vi "in_diff and divided diff.vi"   [LabVIEW 2020, in "NI_Gmath.lvlib"]
uses:
  <vilib>/gmath/NI_Gmath.lvlib
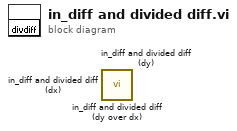
[diagram p0: block diagram]
diagram:
  n1 = call <vilib>:"in_diff and divided diff (dy over dx).vi"() -> ()  [unwired: 15 in, 1 out]
  n2 = call <vilib>:"in_diff and divided diff (dy).vi"() -> ()  [unwired: 15 in, 1 out]
  n3 = call <vilib>:"in_diff and divided diff (dx).vi"() -> ()  [unwired: 15 in, 1 out]
